vi "setAll.vi"(8 "error in (no error)":errorcluster, 10 "MonoSetup":T4, 11 "MonoCommunicator in":refnum<class "MonoCommunicator.lvclass">) -> (0 "error out":errorcluster, 3 "MonoCommunicator out":refnum<class "MonoCommunicator.lvclass">)   [LabVIEW 2020, in "MonoCommunicator.lvclass"]
uses:
  MonoCommunicator.lvclass
  Typedefs/wavelength.ctl
  Typedefs/slitWidth.ctl
  Typedefs/GratingType.ctl
  MonoCommunicator.lvclass/MonoCommunicator.ctl
  MonoPubSubData/MonoPubSubData.lvclass/MonoPubSubData.ctl
  MonoPubSubData/MonoPubSubData.lvclass
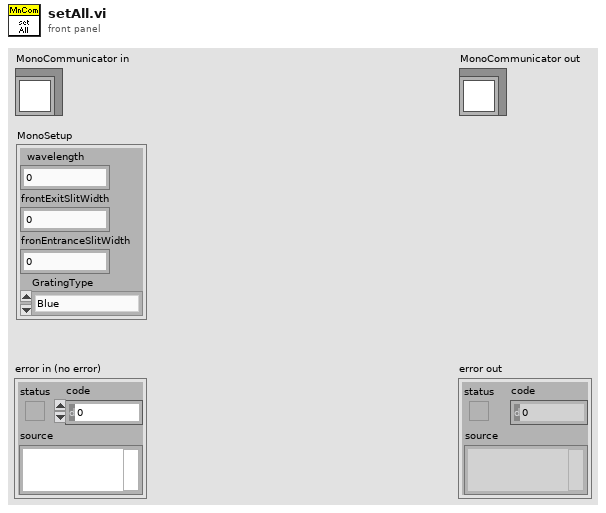
[diagram p1: front panel]
types:
  T1 = typedef "wavelength.ctl" = dbl
  T2 = typedef "slitWidth.ctl" = dbl
  T3 = typedef "GratingType.ctl" = enum16{"Blue", "Red", "Mirror"}
  T4 = cluster{"wavelength":T1, "frontExitSlitWidth":T2, "fronEntranceSlitWidth":T2, "GratingType":T3}
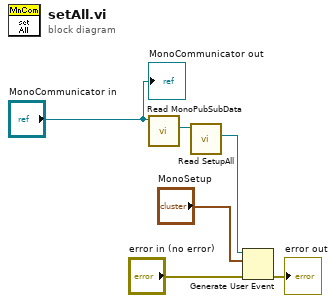
[diagram p0: block diagram]
diagram:
  n1 = call "Read MonoPubSubData.vi"("MonoCommunicator in"="MonoCommunicator in") -> ("MonoPubSubData.lvclass"=w1:refnum<class "MonoPubSubData.lvclass">)  [unwired: 8 in, 2 out]
  n2 = call "Read SetupAll.vi"("MonoPubSubData in"=w1) -> ("SetupAll"=w2:refnum<user-event>)  [unwired: 8 in, 2 out]
  n3 = Generate User Event(user event=w2, event data cluster="MonoSetup", error in="error in (no error)") -> (error out=→"error out":errorcluster)  [unwired: 1 in, 1 out]
  "MonoCommunicator out" <- "MonoCommunicator in"
